vi "PerformStressTests.vi"(2 "error in":errorcluster, 3 "linear actuator info":T1={"distance mm"=100, "Direction"=FALSE, "device name"="Dev2", "speed (mm/s)"=0, "pulse/rev"=400} {"pulse/rev" items=["400"=400, "800"=800, "1600"=1600, "3200"=3200, "6400"=6400, "12800"=12800, "25600"=25600]; "speed (mm/s)" scale=0.0..49.0}, 4 "Test Info":T3={"SD"=0, "Delay"=0.0, "Speed"=0, "Iters"=0, "Type"=enum."OFF", "timeout"=1000}) -> (0 "error out":errorcluster, 1 "mm/s (timed)":dbl)   [LabVIEW 2012]
uses:
  stressTestTypeDef.ctl
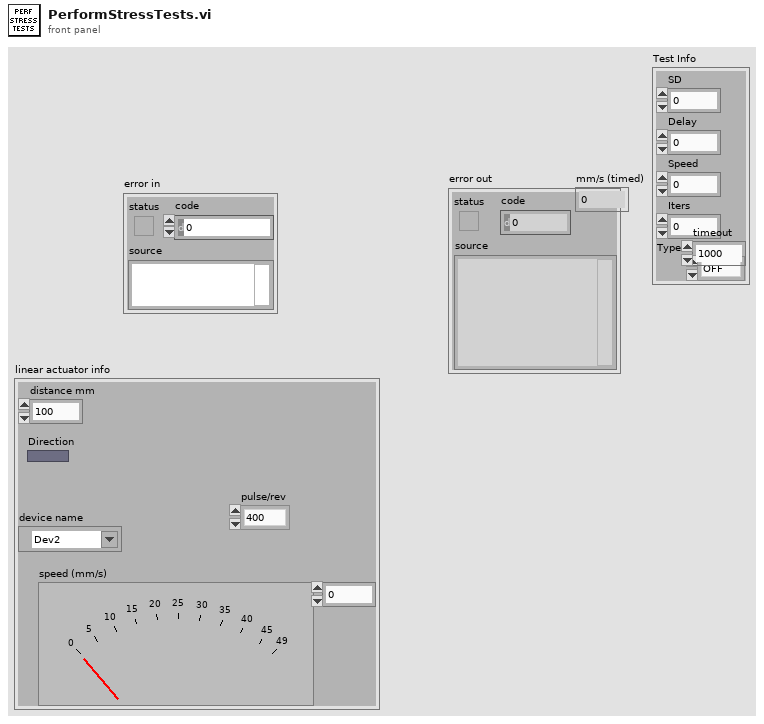
[diagram p1: front panel]
types:
  T1 = cluster{"distance mm":i32, "Direction":bool, "device name":tag, "speed (mm/s)":i32, "pulse/rev":u16}
  T2 = typedef "stressTestTypeDef.ctl" = enum16{"OFF", "ON", "EXTEND", "SPRING", "FRACT ON", "SAC", "FRACT SAC"}
  T3 = cluster{"SD":i32, "Delay":dbl, "Speed":i32, "Iters":i32, "Type":T2, "timeout":i32}
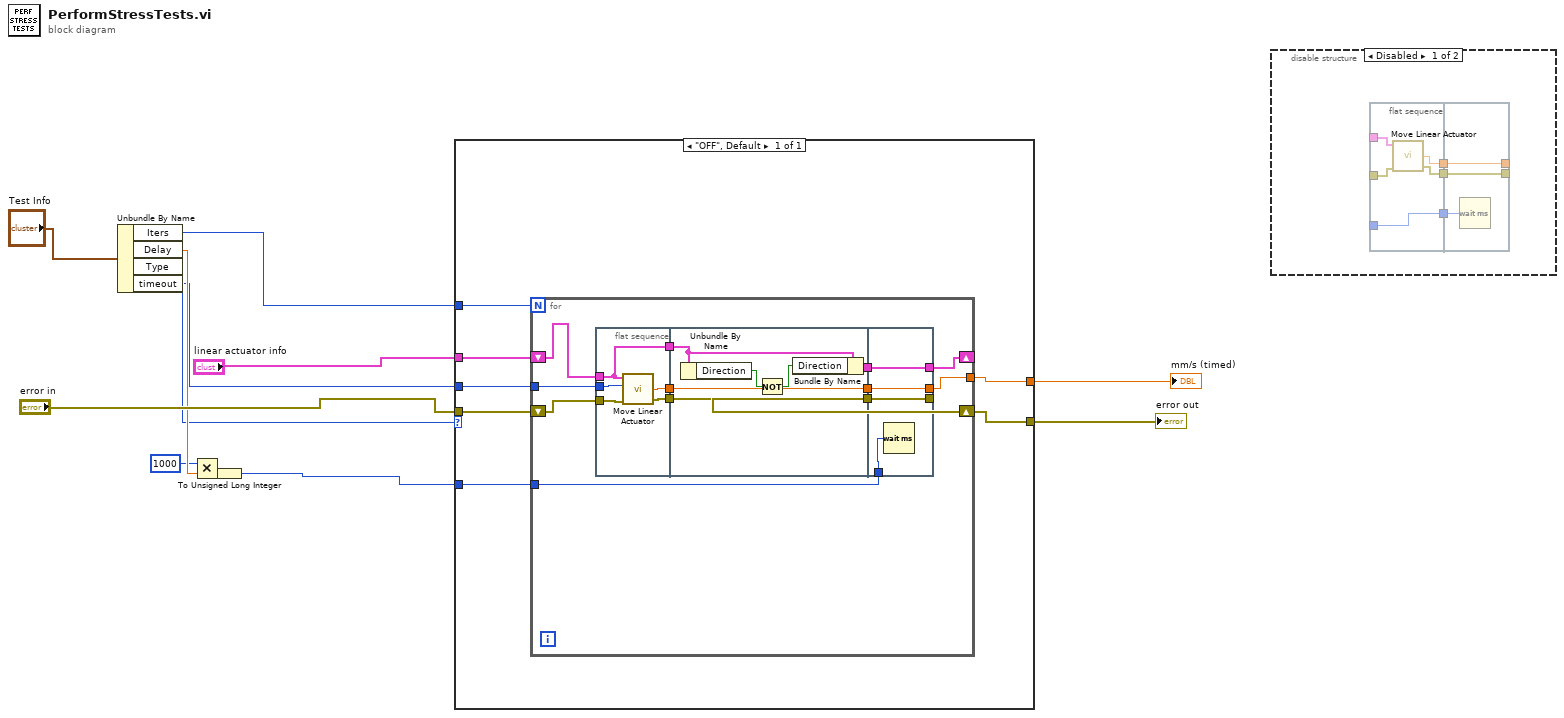
[diagram p0: block diagram]
diagram:
  n1 = Unbundle By Name("Test Info") -> ("Iters"=w8:i32, "Delay"=w7:dbl, "Type"=w3:T2, "timeout"=w2:i32)
  n2 = Multiply(x=1000, y=w7) -> (x*y=w6:dbl)
  n3 = To Unsigned Long Integer(number=w6) -> (unsigned 32bit integer=w4:u32)
  n4 = case shown="\"OFF\", Default" w3 {
    tunnel: [w19] -> w12
    tunnel: [w18] -> w11
    tunnel: "linear actuator info" -> [w17]
    tunnel: "error in" -> [w16]
    tunnel: w8 -> [w15]
    tunnel: w4 -> [w14]
    tunnel: w2 -> [w13]
    frame "OFF", Default {
      n5 = for {
        N: w15 -> [_]
        tunnel: [w32] -> w19
        shift-right: [w31] -> w18
        shift-left: w16 -> [w30]
        shift-right: [w27] -> _
        shift-left: w17 -> [w22]
        tunnel: w14 -> [w23]
        tunnel: w13 -> [w20]
        n6 = flat-sequence {
          tunnel: w30 -> [w35]
          tunnel: [w37] -> w29
          tunnel: [w36] -> w28
          tunnel: w22 -> [w34]
          tunnel: [w34] -> w21
          tunnel: w20 -> [w33]
          tunnel: w29 -> [w43]
          tunnel: w28 -> [w42]
          tunnel: [w43] -> w26
          tunnel: [w42] -> w25
          tunnel: [w41] -> w24
          tunnel: w21 -> [w38]
          tunnel: [w45] -> w27
          tunnel: [w46] -> w31
          tunnel: [w47] -> w32
          tunnel: w26 -> [w47]
          tunnel: w25 -> [w46]
          tunnel: w24 -> [w45]
          tunnel: w23 -> [w44]
          frame #0 {
            n7 = call "Move Linear Actuator.vi"("error in"=w35, "timeout"=w33, "linear actuator info"=w34) -> ("error out"=w36:errorcluster, "mm/s (timed)"=w37:dbl)  [unwired: 1 in, 1 out]
          }
          frame #1 {
            n8 = Unbundle By Name(w38) -> ("Direction"=w40:bool)
            n9 = Not(x=w40) -> (.not. x?=w39:bool)
            n10 = Bundle By Name(cluster=w38, "Direction"=w39) -> (w41:T1)
          }
          frame #2 {
            n11 = Wait (ms)(milliseconds to wait=w44) -> ()  [unwired: 1 out]
          }
        }
      }
    }
  }
  "error out" <- w11
  "mm/s (timed)" <- w12
  n12 = disable-structure shown="Disabled" {
    frame Disabled {
      n13 = flat-sequence {
        tunnel: [w56] -> w48
        tunnel: [w55] -> w51
        tunnel: [w54] -> w50
        tunnel: _ -> [w53]
        tunnel: [w53] -> w49
        tunnel: _ -> [w52]
        tunnel: [w58] -> _
        tunnel: [w59] -> _
        tunnel: w51 -> [w59]
        tunnel: w50 -> [w58]
        tunnel: w49 -> [w57]
        frame #0 {
          n14 = call "Move Linear Actuator.vi"("error in"=w56, "linear actuator info"=w52) -> ("error out"=w54:errorcluster, "mm/s (timed)"=w55:dbl)  [unwired: 2 in, 1 out]
        }
        frame #1 {
          n15 = Wait (ms)(milliseconds to wait=w57) -> ()  [unwired: 1 out]
        }
      }
    }
    frame Enabled {
    }
  }
